vi "InsertItem.vi"(7 "Parent Tag":string, 8 "error in (no error)":errorcluster, 10 "MenuItem":refnum<class "MGI_MenuItem.lvclass">, 11 "Menu in":refnum<class "MGI_ToolStrip.lvclass">) -> (0 "error out":errorcluster, 3 "Menu out":refnum<class "MGI_ToolStrip.lvclass">)   [LabVIEW 2019, in "MGI_ToolStrip.lvclass"]
doc: "Inserts a menu item into the menu.\n\nAuthored by Derek E. Trepanier\nsupport@mooregoodideas.com\nwww.mooregoodideas.com\n\nCopyright (c) 2012, Moore Good Ideas, Inc.\n\nAll rights reserved.\n\nRedistribution and use in source and binary forms, with or without modification, are permitted provided that the following conditions are met:\n\n * Redistributions of source code must retain the above copyright notice, this list of conditions and the following disclaimer.\n * Redistributions in binary form must reproduce the above copyright notice, this list of conditions and the following disclaimer in the documentation and/or other materials provided with the distribution.\n * Neither the name of Moore Good Ideas, Inc. nor the names of its contributors may be used to endorse or promote products derived from this software without specific prior written permission.\n\nTHIS SOFTWARE IS PROVIDED BY THE COPYRIGHT HOLDERS AND CONTRIBUTORS \"AS IS\" AND ANY EXPRESS OR IMPLIED WARRANTIES, INCLUDING, BUT NOT LIMITED TO, THE IMPLIED WARRANTIES OF MERCHANTABILITY AND FITNESS FOR A PARTICULAR PURPOSE ARE DISCLAIMED. IN NO EVENT SHALL THE COPYRIGHT OWNER OR CONTRIBUTORS BE LIABLE FOR ANY DIRECT, INDIRECT, INCIDENTAL, SPECIAL, EXEMPLARY, OR CONSEQUENTIAL DAMAGES (INCLUDING, BUT NOT LIMITED TO, PROCUREMENT OF SUBSTITUTE GOODS OR SERVICES; LOSS OF USE, DATA, OR PROFITS; OR BUSINESS INTERRUPTION) HOWEVER CAUSED AND ON ANY THEORY OF LIABILITY, WHETHER IN CONTRACT, STRICT LIABILITY, OR TORT (INCLUDING NEGLIGENCE OR OTHERWISE) ARISING IN ANY WAY OUT OF THE USE OF THIS SOFTWARE, EVEN IF ADVISED OF THE POSSIBILITY OF SUCH DAMAGE."
uses:
  MGI_ToolStrip.lvclass
  <userlib>/_MGI/Menu Building/MenuItem/MGI_MenuItem.lvclass
  System.Windows.Forms
  MGI_ToolStrip.lvclass/MGI_ToolStrip.ctl
  <userlib>/_MGI/Menu Building/MenuItem/Read Enabled.vi
  <userlib>/_MGI/Menu Building/MenuItem/Read Full Tag.vi
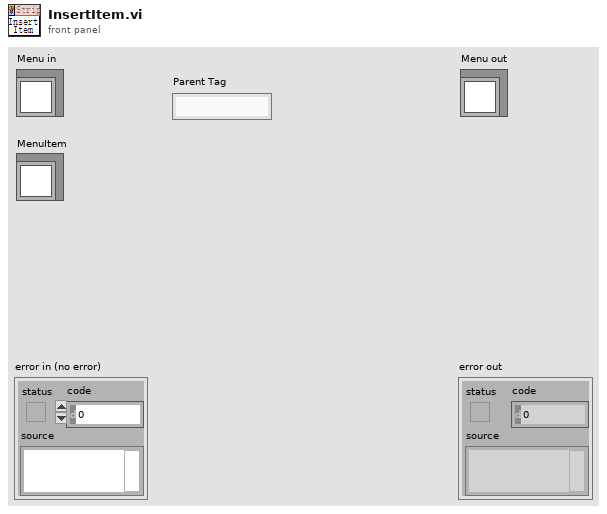
[diagram p1: front panel]
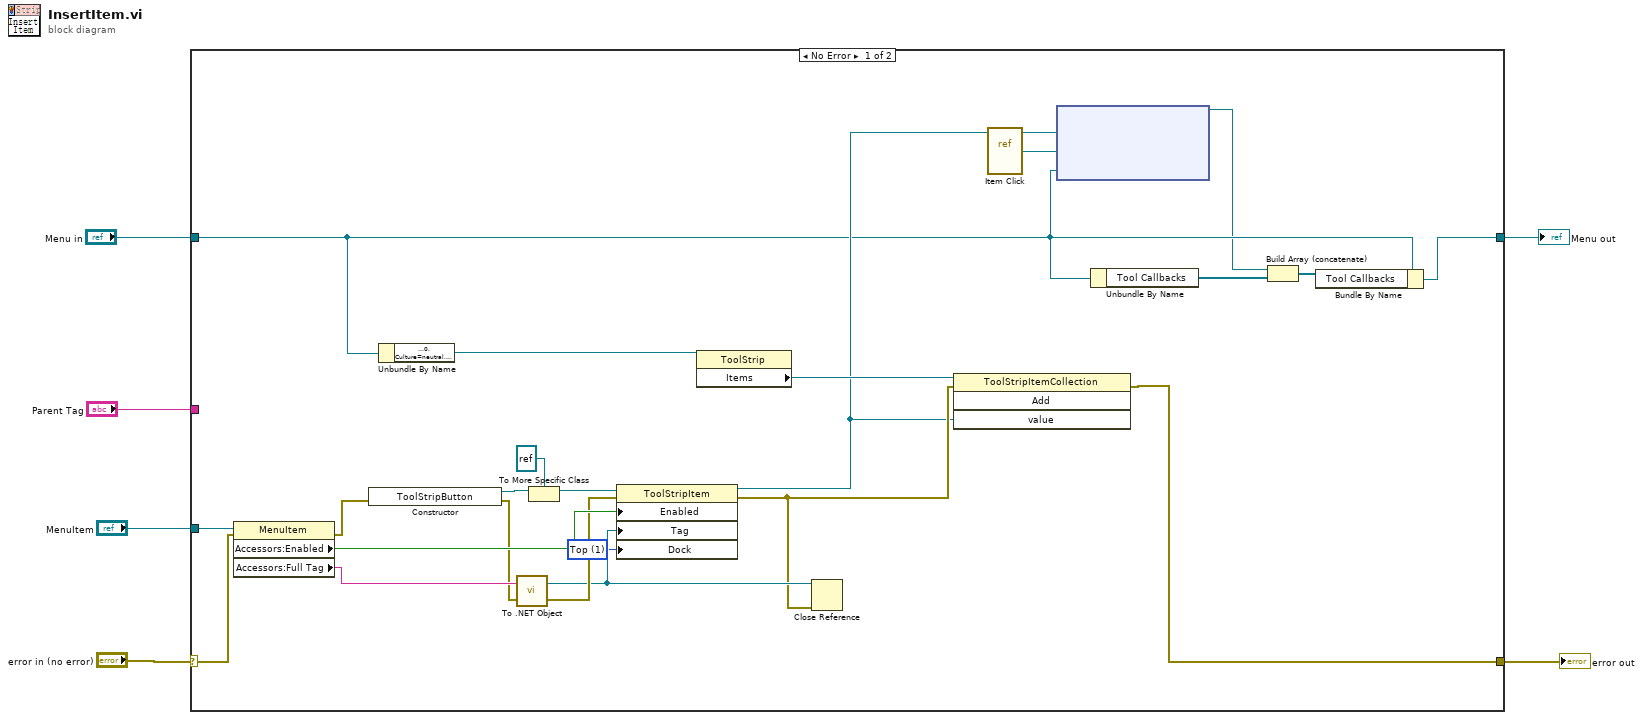
[diagram p0: block diagram]
diagram:
  n1 = case shown="No Error" "error in (no error)" {
    selector: "error in (no error)" -> [w9 w30]
    tunnel: "Menu in" -> [w16 w31]
    tunnel: [w14 w31] -> w5
    tunnel: [w8 w30] -> w3
    tunnel: "MenuItem" -> [w29 _]
    tunnel: "Parent Tag" -> [_ _]
    frame No Error {
      w7 = 1 items=["None", "Top", "Bottom", "Left", "Right", "Fill"] ("Dock")
      n2 = property class="MenuItem"(reference=w29, error in=w9) -> (error out=w10:errorcluster, "Accessors:Enabled"=w25:bool, "Accessors:Full Tag"=w24:string)  [unwired: 1 out]
      n3 = constructor class="ToolStripButton"(error in=w10) -> (reference out=w27:refnum<k24>, error out=w23:errorcluster)  [unwired: 2 in, 1 out]
      n4 = Unbundle By Name(w16) -> ("ToolStrip"=w20:refnum<k24>)
      n5 = call <vilib>:"To .NET Object.vi"("error in (no error)"=w23, "anything"=w24) -> ("error out"=w22:errorcluster, ".NET object"=w21:refnum<k24>)
      n6 = To More Specific Class(target class=refnum<k24> refnum ("new reference"), reference=w27) -> (specific class reference=w26:refnum<k24>)  [unwired: 1 in, 1 out]
      n7 = property class="ToolStripItem"(reference=w26, error in=w22, "Enabled"=w25, "Tag"=w21, "Dock"=w7) -> (reference out=w17:refnum<k24>, error out=w18:errorcluster)
      n8 = property class="ToolStrip"(reference=w20) -> ("Items"=w19:refnum<k24>)  [unwired: 1 in, 2 out]
      n9 = Close Reference(reference=w21, error in (no error)=w18) -> ()  [unwired: 1 out]
      n10 = invoke class="ToolStripItemCollection" method="Add"(reference=w19, error in=w18, "value"=w17) -> (error out=w8:errorcluster)  [unwired: 1 in, 3 out]
      n11 = vi-ref "Item Click.vi"() -> ("vi reference"=w11:refnum<vi>)
      n12 = node(w17, w11, w16) -> (w12:refnum<k27>)  [unwired: 2 in, 1 out]
      n13 = Unbundle By Name(w16) -> ("Tool Callbacks"=w15:refnum<k27>[])
      n14 = Build Array (concatenate)(w12, w15) -> (w13:refnum<k27>[])
      n15 = Bundle By Name(cluster=w16, "Tool Callbacks"=w13) -> (w14:refnum<class "MGI_ToolStrip.lvclass">)
    }
    frame Error {
    }
  }
  "error out" <- w3
  "Menu out" <- w5
